vi "Solution.vi"() -> ()   [LabVIEW 2020]
panel:
  out "result":u64
  in  "data?":bool
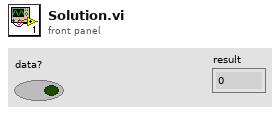
[diagram p1: front panel]
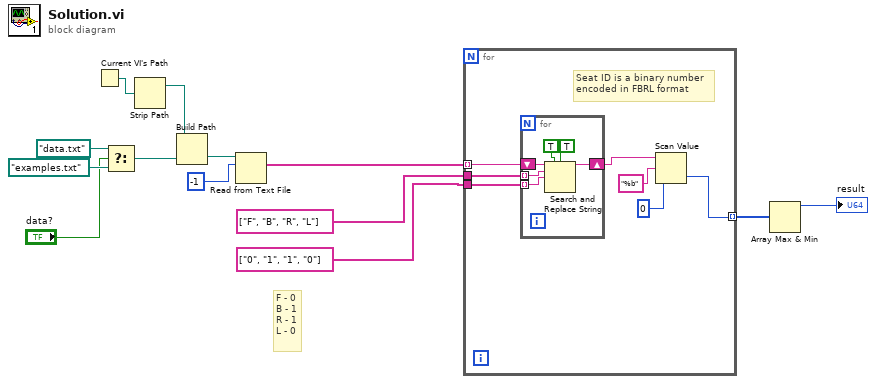
[diagram p0: block diagram]
diagram:
  # "F - 0\nB - 1\nR - 1\nL - 0"
  n1 = Current VI's Path() -> (path=w9:path)
  n2 = Select(t=path "data.txt", s="data?", f=path "examples.txt") -> (s? t:f=w10:path)
  n3 = Strip Path(path=w9) -> (stripped path=w8:path)  [unwired: 1 out]
  n4 = Build Path(base path=w8, name or relative path=w10) -> (appended path=w7:path)
  n5 = Read from Text File(file (use dialog)=w7, count=-1) -> (text=w4:string[])  [unwired: 2 in, 3 out]
  n6 = for {
    tunnel: w4 -> [w20] mode=indexing
    tunnel: [w15] -> w6 mode=indexing
    tunnel: string[] ["F", "B", "R", "L"] -> [w19]
    tunnel: string[] ["0", "1", "1", "0"] -> [w18]
    # "Seat ID is a binary number\nencoded in FBRL format"
    n7 = for {
      shift-right: [w25] -> w16
      shift-left: w20 -> [w26]
      tunnel: w19 -> [w24] mode=indexing
      tunnel: w18 -> [w23] mode=indexing
      n8 = Search and Replace String(replace all?=TRUE ("replace all? (F)"), case sensitive?=TRUE ("ignore case? (F)"), input string=w26, search string=w24, replace string=w23) -> (result string=w25:string)  [unwired: 3 in, 3 out]
    }
    n9 = Scan Value(string=w16, format string="%b", default (0 dbl)=u64 0) -> (value=w15:u64)  [unwired: 1 out]
  }
  n10 = Array Max & Min(array=w6) -> (max value=→"result":u64)  [unwired: 3 out]
